vi "TDMS(Close).vi"(8 "error in (no error)":errorcluster caption="错误输入（无错误）", 11 "tdms文件":refnum<k34>) -> (0 "error out":errorcluster caption="错误输出")   [LabVIEW 2020, in "人体健康监测系统.lvclass"]
uses:
  e9e87d26-3e84-4e6a-964a-aa8ff9d0bb5a.vi
  e7740419-0e76-41c7-a585-d67317e1485a.vi
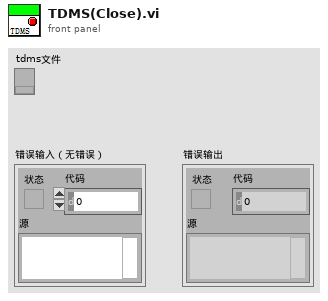
[diagram p1: front panel]
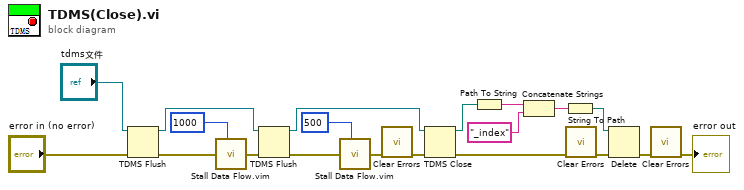
[diagram p0: block diagram]
diagram:
  n1 = TDMS Flush(4:"error in (no error)", 7:"tdms文件") -> (0:w7:errorcluster, 3:w9:refnum<k34>)
  n2 = call "Stall Data Flow.vim"("value in"=w7, "milliseconds to wait"=u32 1000) -> ("value out"=w5:errorcluster)  [unwired: 1 out]
  n3 = TDMS Flush(4:w5, 7:w9) -> (0:w6:errorcluster, 3:w8:refnum<k34>)
  n4 = call "Stall Data Flow.vim"("value in"=w6, "milliseconds to wait"=u32 500) -> ("value out"=w11:errorcluster)  [unwired: 1 out]
  n5 = call <vilib>:"Clear Errors.vi"("error in (no error)"=w11) -> ("error out"=w12:errorcluster)  [unwired: 5 in, 1 out]
  n6 = TDMS Close(8:w12, 11:w8) -> (0:w14:errorcluster, 3:w20:path)
  n7 = Path To String(path=w20) -> (string=w19:string)
  n8 = Concatenate Strings(w19, "_index") -> (w17:string)
  n9 = String To Path(string=w17) -> (path=w13:path)
  n10 = call <vilib>:"Clear Errors.vi"("error in (no error)"=w14) -> ("error out"=w15:errorcluster)  [unwired: 5 in, 1 out]
  n11 = Delete(path (use dialog)=w13, error in=w15) -> (error out=w16:errorcluster)  [unwired: 3 in, 2 out]
  n12 = call <vilib>:"Clear Errors.vi"("error in (no error)"=w16) -> ("error out"=→"error out":errorcluster)  [unwired: 5 in, 1 out]
